vi "worksheet set paper.vi"(8 "error in (no error)":errorcluster, 10 "paper_type":u8, 11 "worksheet":u32) -> (0 "error out":errorcluster)   [LabVIEW 2015, in "xlsxwriter.lvlib"]
doc: "void worksheet_set_paper(lxw_worksheet worksheet, uint8_t paper_type);"
uses:
  xlsxwriter.lvlib
  xlsxwriter.dll
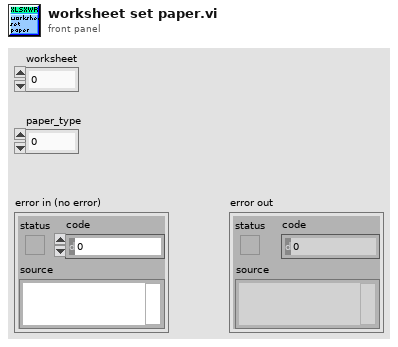
[diagram p1: front panel]
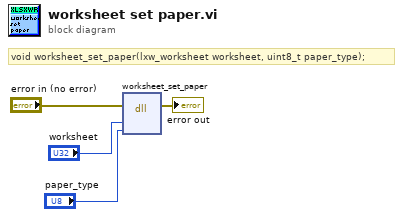
[diagram p0: block diagram]
diagram:
  # "void worksheet_set_paper(lxw_worksheet worksheet, uint8_t paper_type);"
  n1 = dll-call lib="C:/Users/WDAGUtilityAccount/Desktop/lv_vis_added_cell/xlsxwriter.*" fn="worksheet_set_paper"(error in="error in (no error)", "worksheet"="worksheet", "paper_type"="paper_type") -> (error out=→"error out":errorcluster)  [unwired: 5 in, 1 out]
